vi "Set Voltage and Current.vi"(0 "Yokogawa WT500 in":refnum<class "Yokogawa WT500.lvclass">, 5 "Card #":u8, 7 "Voltage enum number":u16, 9 "Current enum number":u16, 11 "error in (no error)":errorcluster) -> (4 "Yokogawa WT500 out":refnum<class "Yokogawa WT500.lvclass">, 15 "error out":errorcluster)   [LabVIEW 2014, in "Generic Power Analyzer.lvlib" / "Yokogawa WT500.lvlib" / "Yokogawa WT500.lvclass"]
uses:
  Yokogawa WT500.lvclass
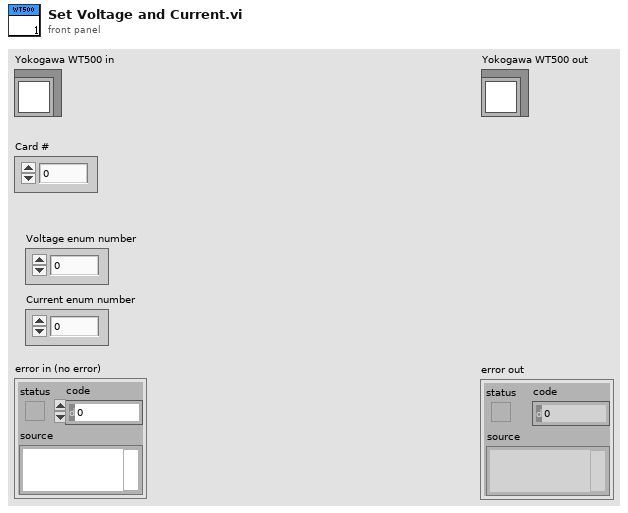
[diagram p1: front panel]
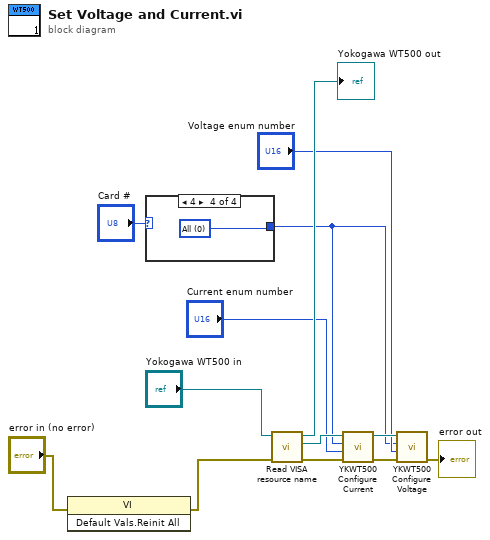
[diagram p0: block diagram]
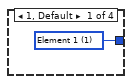
[diagram p2: hidden frame]
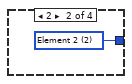
[diagram p3: hidden frame]
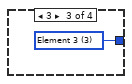
[diagram p4: hidden frame]
diagram:
  n1 = invoke class="VI" method="Default Vals.Reinit All"(error in="error in (no error)") -> (error out=w1:errorcluster)  [unwired: 2 in, 2 out]
  n2 = case shown="4" "Card #" {
    tunnel: [w14 w15 w16 w17] -> w3
    frame 1, Default {
      w14 = u16 1 items=["All", "Element 1", "Element 2", "Element 3", "Sigma"] ("Element (0: All)")
    }
    frame 2 {
      w15 = u16 2 items=["All", "Element 1", "Element 2", "Element 3", "Sigma"] ("Element (0: All)")
    }
    frame 3 {
      w16 = u16 3 items=["All", "Element 1", "Element 2", "Element 3", "Sigma"] ("Element (0: All)")
    }
    frame 4 {
      w17 = u16 0 items=["All", "Element 1", "Element 2", "Element 3", "Sigma"] ("Element (0: All)")
    }
  }
  n3 = call-dynamic "Read VISA resource name.vi"("error in (no error)"=w1, "Generic Instrument in"="Yokogawa WT500 in") -> ("error out"=w8:errorcluster, "VISA resource name"=w9:refnum<visa-resource-name>, "Generic Instrument out"=→"Yokogawa WT500 out":refnum<class "Yokogawa WT500.lvclass">)  [unwired: 7 in]
  n4 = call <instrlib>:"YKWT500 Configure Current.vi"("error in (no error)"=w8, "Current Range (7: 40A)"="Current enum number", "Element (0: All)"=w3, "VISA resource name"=w9) -> ("error out"=w11:errorcluster, "VISA resource name out"=w10:refnum<visa-resource-name>)  [unwired: 6 in]
  n5 = call <instrlib>:"YKWT500 Configure Voltage.vi"("error in (no error)"=w11, "Voltage Range (8: 1000V)"="Voltage enum number", "Element (0: All)"=w3, "VISA resource name"=w10) -> ("error out"=→"error out":errorcluster)  [unwired: 6 in, 1 out]
